vi "PID-Regler.vi"(6 "ECO Mode":bool, 7 "Regler EIN":bool=TRUE, 8 "Output Range":cluster{"Output High":sgl, "Output Low":sgl}, 9 "PID-Parameter":T1, 10 "Istwert":sgl, 11 "Sollwert":sgl) -> (1 "Output":i16)   [LabVIEW 2020, in "Regler.lvlib"]
uses:
  Regler.lvlib
  <vilib>/addons/control/pid/pid.llb/PID (DBL).vi
  <vilib>/addons/control/pid/NI_PID_pid.lvlib
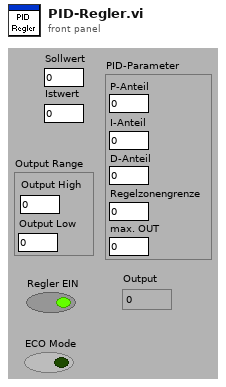
[diagram p1: front panel]
types:
  T1 = cluster{"P-Anteil":sgl, "I-Anteil":sgl, "D-Anteil":sgl, "Regelzonengrenze":sgl, "max. OUT":sgl}
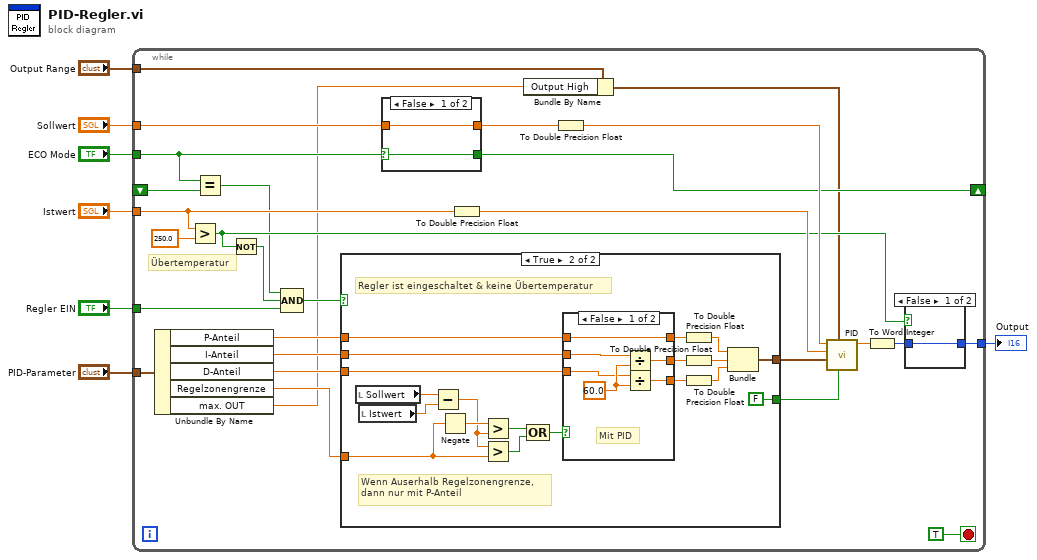
[diagram p0: block diagram]
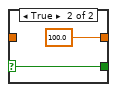
[diagram p2: hidden frame]
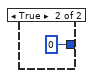
[diagram p3: hidden frame]
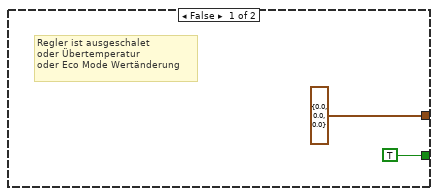
[diagram p4: hidden frame]
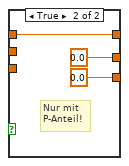
[diagram p5: hidden frame]
diagram:
  n1 = while {
    tunnel: "PID-Parameter" -> [w11]
    tunnel: "Output Range" -> [w10]
    tunnel: "Istwert" -> [w31]
    tunnel: "Regler EIN" -> [w29]
    tunnel: [w25] -> w3
    tunnel: "Sollwert" -> [w18]
    tunnel: "ECO Mode" -> [w13]
    shift-right: [w15] -> _
    shift-left: _ -> [w14]
    stop <- TRUE stop-if-true
    # "Übertemperatur"
    n2 = Unbundle By Name(w11) -> ("P-Anteil"=w23:sgl, "I-Anteil"=w22:sgl, "D-Anteil"=w21:sgl, "Regelzonengrenze"=w19:sgl, "max. OUT"=w8:sgl)
    n3 = Greater?(x=w31, y=sgl 250.0) -> (0:w24:bool)
    n4 = Equal?(x=w13, y=w14) -> (x = y?=w12:bool)
    n5 = Not(x=w24) -> (.not. x?=w27:bool)
    n6 = Compound Arithmetic op=AND(w12, w27, w29) -> (w28:bool)
    n7 = case shown="True" w28 {
      tunnel: [cluster{dbl, dbl, dbl} {0.0, 0.0, 0.0} w59] -> w32
      tunnel: w23 -> [_ w58]
      tunnel: w22 -> [_ w57]
      tunnel: w21 -> [_ w56]
      tunnel: [TRUE FALSE] -> w20
      tunnel: w19 -> [_ w44]
      frame False {
        # "Regler ist ausgeschalet\noder Übertemperatur\noder Eco Mode Wertänderung"
      }
      frame True {
        # "Wenn Auserhalb Regelzonengrenze,\ndann nur mit P-Anteil"
        # "Regler ist eingeschaltet & keine Übertemperatur"
        n8 = local read "Sollwert"() -> (w47:sgl)
        n9 = local read "Istwert"() -> (w46:sgl)
        n10 = Subtract(x=w47, y=w46) -> (x-y=w48:sgl)
        n11 = Negate(x=w44) -> (-x=w49:sgl)
        n12 = Greater?(x=w49, y=w48) -> (0:w50:bool)
        n13 = Greater?(x=w48, y=w44) -> (0:w51:bool)
        n14 = Compound Arithmetic op=OR(w50, w51) -> (w45:bool)
        n15 = case shown="False" w45 {
          tunnel: w58 -> [w65 w71]
          tunnel: w57 -> [w67 _]
          tunnel: w56 -> [w66 _]
          tunnel: [w65 w71] -> w55
          tunnel: [w64 sgl 0.0] -> w54
          tunnel: [w63 sgl 0.0] -> w53
          frame False {
            w68 = sgl 60.0 ("y")
            # "Mit PID"
            n16 = Divide(x=w67, y=w68) -> (x/y=w64:sgl)
            n17 = Divide(x=w66, y=w68) -> (x/y=w63:sgl)
          }
          frame True {
            # "Nur mit \nP-Anteil!"
          }
        }
        n18 = To Double Precision Float(number=w55) -> (double precision float=w60:dbl)
        n19 = To Double Precision Float(number=w54) -> (double precision float=w61:dbl)
        n20 = To Double Precision Float(number=w53) -> (double precision float=w62:dbl)
        n21 = Bundle(w60, w61, w62) -> (w59:cluster{dbl, dbl, dbl})  [unwired: 1 in]
      }
    }
    n22 = case shown="False" w13 {
      selector: w13 -> [w36 w38]
      tunnel: w18 -> [w37 _]
      tunnel: [w37 sgl 100.0 ("Sollwert")] -> w17
      tunnel: [w36 w38] -> w15
      frame False {
      }
      frame True {
      }
    }
    n23 = To Double Precision Float(number=w31) -> (double precision float=w34:dbl)
    n24 = Bundle By Name(cluster=w10, "Output High"=w8) -> (w9:cluster{"Output High":sgl, "Output Low":sgl})
    n25 = To Double Precision Float(number=w17) -> (double precision float=w33:dbl)
    n26 = call-poly <vilib>:"PID.vi"("reinitialize? (F)"=w20, "output range"=w9, "PID gains"=w32, "process variable"=w34, "setpoint"=w33) -> ("output"=w35:dbl)  [unwired: 5 in, 1 out]
    n27 = To Word Integer(number=w35) -> (16bit integer=w26:i16)
    n28 = case shown="False" w24 {
      tunnel: [w40 i16 0] -> w25
      tunnel: w26 -> [w40 _]
      frame False {
      }
      frame True {
      }
    }
  }
  "Output" <- w3
